vi "Update Message Getter.vi"(7 "RPC Message Name":string, 8 "error in (no error)":errorcluster, 10 "Message Getter in":refnum<vi>, 11 "RPC Messages Folder (ProjectItem) in":refnum<vi>) -> (0 "error out":errorcluster, 2 "Message Getter out":refnum<vi>, 3 "RPC Messages Folder (ProjectItem) out":refnum<vi>)   [LabVIEW 2019, in "gRPC Template Creation Utility.lvlib"]
uses:
  gRPC Template Creation Utility.lvlib
  <vilib>/Utility/traverseref.llb/VI Scripting - Traverse.lvlib
  <vilib>/Utility/traverseref.llb/TRef TravTarget.ctl
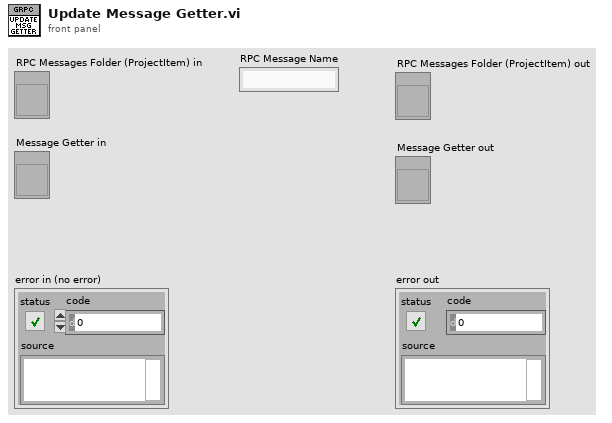
[diagram p1: front panel]
types:
  T1 = typedef "TRef TravTarget.ctl" = enum16{"FP", "BD", "Other"}
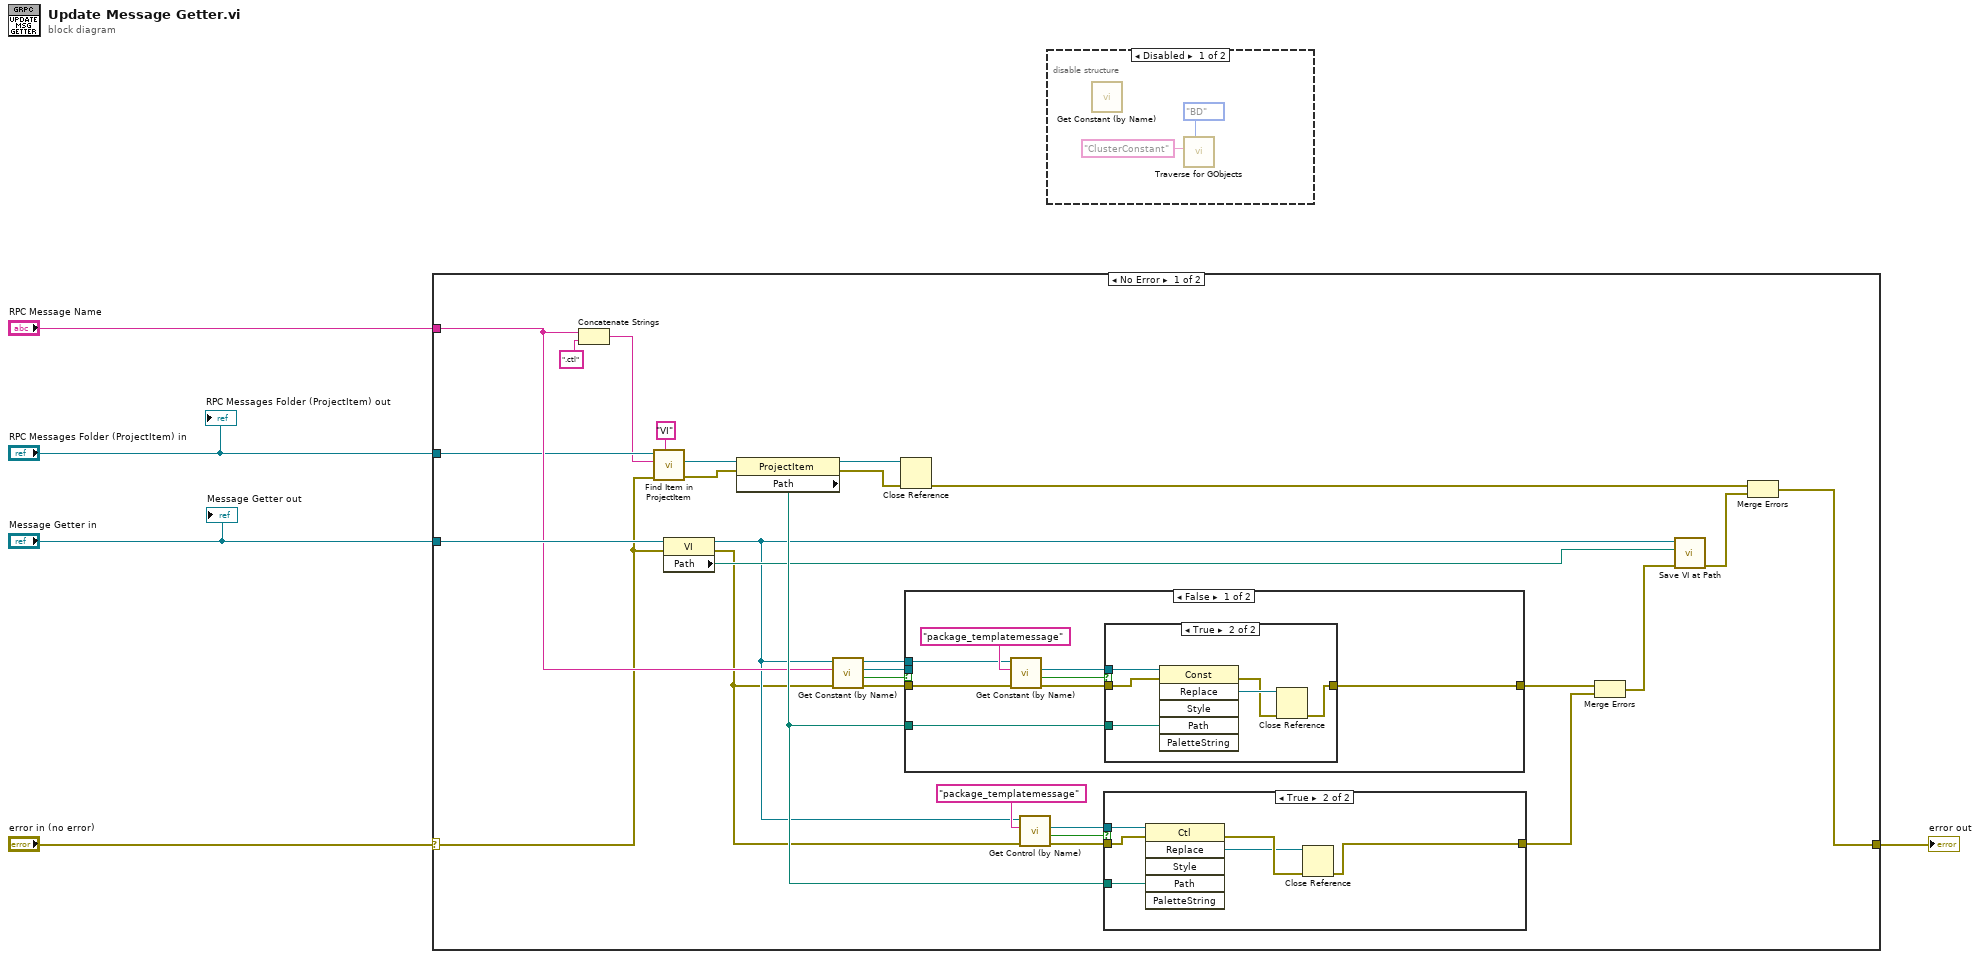
[diagram p0: block diagram]
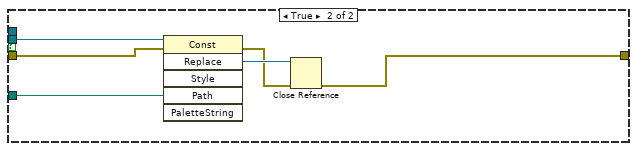
[diagram p4: hidden frame]
diagram:
  n1 = case shown="No Error" "error in (no error)" {
    selector: "error in (no error)" -> [w18 w63]
    tunnel: "Message Getter in" -> [w29 _]
    tunnel: [w28 w63] -> w4
    tunnel: "RPC Message Name" -> [w21 _]
    tunnel: "RPC Messages Folder (ProjectItem) in" -> [w19 _]
    frame No Error {
      n2 = Concatenate Strings(w21, ".ctl" ("string")) -> (w13:string)
      n3 = call "Find Item in ProjectItem.vi"("Item Type"="VI", "error in (no error)"=w18, "Name"=w13, "ProjectItem in"=w19) -> ("error out"=w23:errorcluster, "Item Refnum out"=w22:refnum<vi>)  [unwired: 4 in, 2 out]
      n4 = property class="VI"(reference=w29, error in=w18) -> (reference out=w9:refnum<vi>, error out=w8:errorcluster, "Path"=w30:path)
      n5 = property class="ProjectItem"(reference=w22, error in=w23) -> (reference out=w24:refnum<vi>, error out=w25:errorcluster, "Path"=w31:path)
      n6 = call "Get Constant (by Name).vi"("error in (no error)"=w8, "Constant Label"=w21, "Owner VI in"=w9) -> ("error out"=w11:errorcluster, "Found ?"=w7:bool, "Const ref out"=w6:refnum<vi>, "Owner VI out"=w10:refnum<vi>)  [unwired: 5 in]
      n7 = Close Reference(reference=w24, error in (no error)=w25) -> (error out=w27:errorcluster)
      n8 = case shown="False" w7 {
        tunnel: [w42 w50] -> w32
        tunnel: w31 -> [w41 w51]
        tunnel: w11 -> [w36 w55]
        tunnel: w10 -> [w35 _]
        tunnel: w6 -> [_ w54]
        frame False {
          n9 = call "Get Constant (by Name).vi"("error in (no error)"=w36, "Constant Label"="package_templatemessage" ("name/order"), "Owner VI in"=w35) -> ("error out"=w38:errorcluster, "Found ?"=w37:bool, "Const ref out"=w40:refnum<vi>)  [unwired: 5 in, 1 out]
          n10 = case shown="True" w37 {
            tunnel: [w43 w49] -> w42
            tunnel: w41 -> [_ w48]
            tunnel: w40 -> [_ w45]
            tunnel: w38 -> [w43 w44]
            frame False {
            }
            frame True {
              n11 = invoke class="Const" method="Replace"(reference=w45, error in=w44, "Path"=w48) -> (error out=w46:errorcluster, "Replace"=w47:refnum<vi>)  [unwired: 3 in, 4 out]
              n12 = Close Reference(reference=w47, error in (no error)=w46) -> (error out=w49:errorcluster)
            }
          }
        }
        frame True {
          n13 = invoke class="Const" method="Replace"(reference=w54, error in=w55, "Path"=w51) -> (error out=w52:errorcluster, "Replace"=w53:refnum<vi>)  [unwired: 3 in, 4 out]
          n14 = Close Reference(reference=w53, error in (no error)=w52) -> (error out=w50:errorcluster)
        }
      }
      n15 = call "Get Control (by Name).vi"("error in (no error)"=w8, "Control Label"="package_templatemessage" ("name/order"), "Owner VI in"=w9) -> ("error out"=w15:errorcluster, "Found ?"=w12:bool, "Control Refnum"=w16:refnum<vi>)  [unwired: 5 in, 1 out]
      n16 = case shown="True" w12 {
        tunnel: [w56 w62] -> w33
        tunnel: w31 -> [_ w59]
        tunnel: w16 -> [_ w58]
        tunnel: w15 -> [w56 w57]
        frame False {
        }
        frame True {
          n17 = invoke class="Ctl" method="Replace"(reference=w58, error in=w57, "Path"=w59) -> (error out=w61:errorcluster, "Replace"=w60:refnum<vi>)  [unwired: 3 in, 4 out]
          n18 = Close Reference(reference=w60, error in (no error)=w61) -> (error out=w62:errorcluster)
        }
      }
      n19 = Merge Errors(w32, w33) -> (w34:errorcluster)
      n20 = call "Save VI at Path.vi"("error in (no error)"=w34, "Path"=w30, "VI in"=w9) -> ("error out"=w26:errorcluster)  [unwired: 6 in, 2 out]
      n21 = Merge Errors(w27, w26) -> (w28:errorcluster)
    }
    frame Error {
    }
  }
  "error out" <- w4
  n22 = disable-structure shown="Disabled" {
    frame Disabled {
      n23 = call "Get Constant (by Name).vi"() -> ()  [unwired: 8 in, 4 out]
      n24 = call <vilib>:"Traverse for GObjects.vi"("Traverse Target"=TRef_TravTarget."BD", "Class Name"="ClusterConstant") -> ()  [unwired: 6 in, 4 out]
    }
    frame Enabled {
    }
  }
  "RPC Messages Folder (ProjectItem) out" <- "RPC Messages Folder (ProjectItem) in"
  "Message Getter out" <- "Message Getter in"
